vi "interpolate.vi"(8 "error in (no error)":errorcluster, 11 "Thorcam in":refnum<class "Thorcam.lvclass">) -> (0 "error out":errorcluster, 2 "position out":dbl, 3 "Thorcam out":refnum<class "Thorcam.lvclass">)   [LabVIEW 2012, in "Thorcam.lvclass"]
uses:
  Thorcam.lvclass
  Thorcam.lvclass/Thorcam.ctl
  <vilib>/gmath/NI_Gmath.lvlib
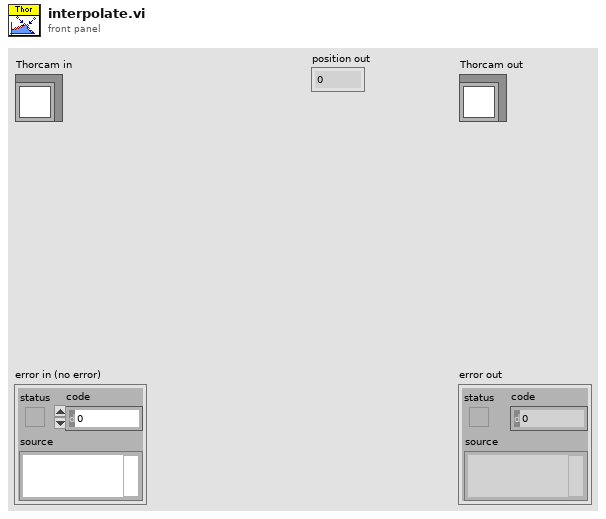
[diagram p1: front panel]
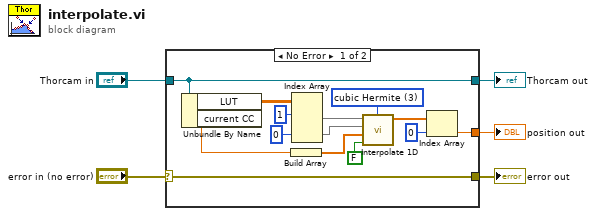
[diagram p0: block diagram]
diagram:
  n1 = case shown="No Error" "error in (no error)" {
    selector: "error in (no error)" -> [w19 w21]
    tunnel: [w19 w21] -> w4
    tunnel: [w18 w20] -> w2
    tunnel: "Thorcam in" -> [w18 w20]
    tunnel: [w8 _] -> w1
    frame No Error {
      w9 = 3 items=["nearest", "linear", "spline", "cubic Hermite", "Lagrange"] ("method")
      n2 = Unbundle By Name(w18) -> ("LUT"=w17:dbl[][], "current CC"=w6:dbl)
      n3 = Build Array(w6) -> (w7:dbl[])
      n4 = Index Array(array=w17, index (row) #1=1 ("index (row)"), index (row) #2=0 ("index (row)")) -> (element #1=w13:dbl[], element #2=w12:dbl[])  [unwired: 2 in]
      n5 = call <vilib>:"Interpolate 1D.vi"("method"=w9, "X is monotonic"=FALSE, "xi"=w7, "X"=w12, "Y"=w13) -> ("yi"=w10:dbl[])  [unwired: 4 in, 2 out]
      n6 = Index Array(array=w10, index=0) -> (element=w8:dbl)
    }
    frame Error {
    }
  }
  "error out" <- w4
  "Thorcam out" <- w2
  "position out" <- w1
